vi "Launch Connection Async.vi"(8 "error in (no error)":errorcluster, 11 "TCP Comm In":T1) -> (0 "error out":errorcluster, 3 "TCP Comm":T1)   [LabVIEW 2020, in "TinyTCP.lvlib"]
uses:
  TinyTCP.lvlib
  Connection Loop.vi
  State.ctl
  Ref Data.ctl
  Instance.ctl
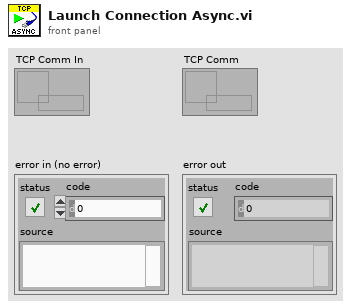
[diagram p1: front panel]
types:
  T1 = typedef "TinyTCP.lvlib/Instance.ctl" = refnum<data-value>
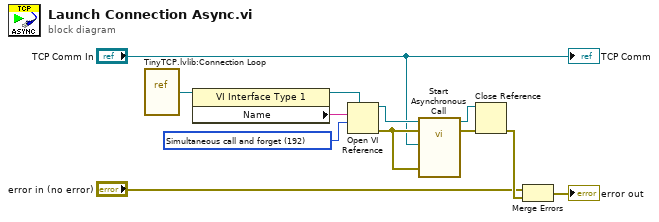
[diagram p0: block diagram]
diagram:
  w7 = 192 items=["Record modifications"=1, "Open templates for editing"=2, "Prompt user to save"=4, "Prepare for reentrant run"=8, "Prompt to find missing subVIs"=16, "Hide loading dialog box"=32, "Enable simultaneous calls"=64, "Prepare to call and forget"=128, "Simultaneous call and forget"=192, "Prepare to call and collect"=256, "Simultaneous call and collect"=320]
  n1 = vi-ref "TinyTCP.lvlib:Connection Loop.vi"() -> (w5:refnum<vi>)
  n2 = property class="VI Interface Type 1"(reference=w5) -> (reference out=w8:refnum<vi>, "Name"=w6:string)  [unwired: 1 in, 1 out]
  n3 = Open VI Reference(type specifier VI Refnum (for type only)=w8, vi path=w6, options=w7) -> (vi reference=w9:refnum<vi>, error out=w12:errorcluster)  [unwired: 3 in]
  n4 = call-by-ref "Start Asynchronous Call"(reference=w9, error in=w12, 8:"error in (no error)"=w12, "TCP Comm"="TCP Comm In") -> (reference out=w11:refnum<vi>, error out=w10:errorcluster)  [unwired: 9 in, 1 out]
  n5 = Close Reference(reference=w11, error in (no error)=w10) -> (error out=w3:errorcluster)
  n6 = Merge Errors("error in (no error)", w3) -> (→"error out":errorcluster)
  "TCP Comm" <- "TCP Comm In"
